vi "SimpleOscilloscopeMain.vi"() -> ()   [LabVIEW 2020]
uses:
  Oscilloscope.lvclass
  Oscilloscope.lvclass/Oscilloscope.ctl
panel:
  out "Waveform Graph":waveform(dbl)[](graph)
  out "error out":errorcluster
  in  "Stop Button":bool
  in  "error in (no error)":errorcluster
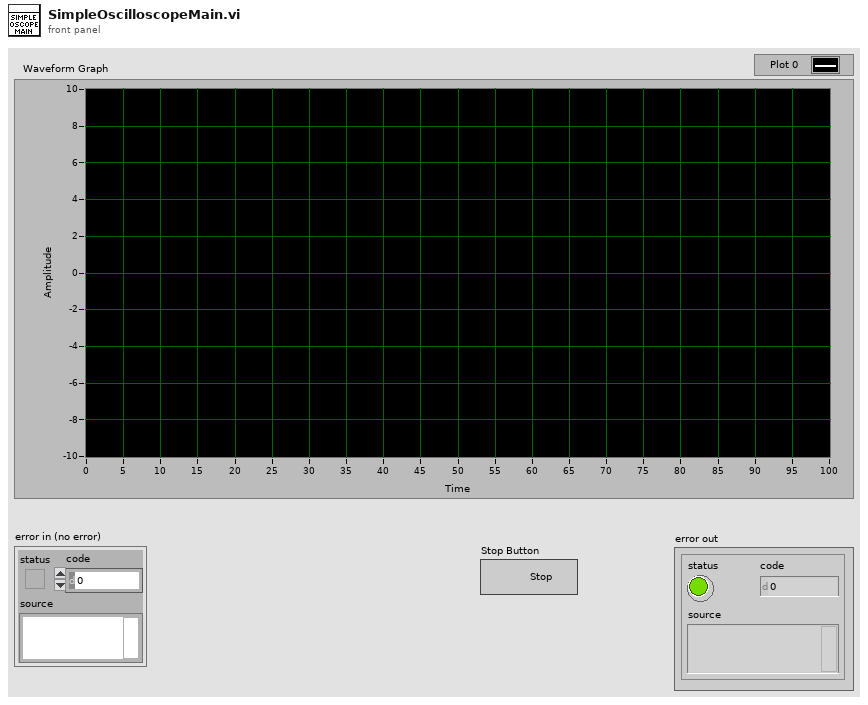
[diagram p1: front panel]
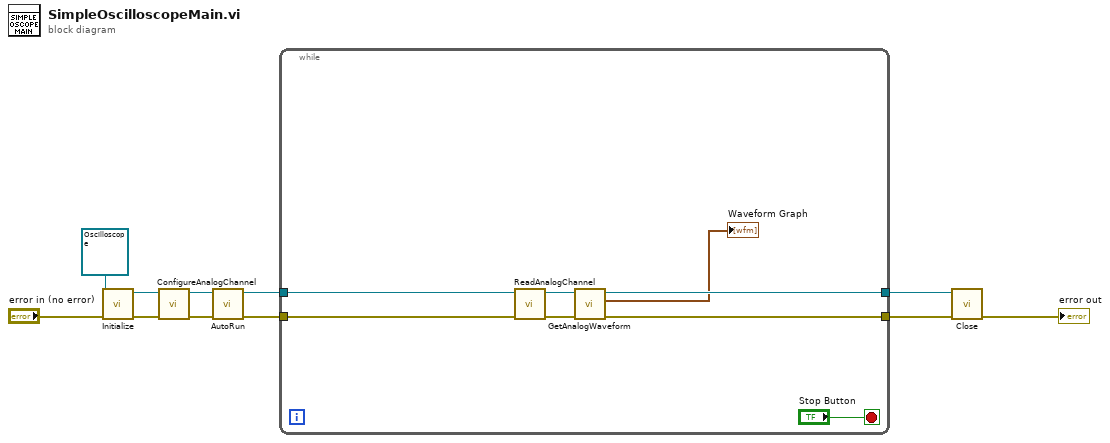
[diagram p0: block diagram]
diagram:
  n1 = call-dynamic "Initialize.vi"("error in (no error)"="error in (no error)", "Oscilloscope in"=refnum<class "Oscilloscope.lvclass"> refnum) -> ("error out"=w9:errorcluster, "Oscilloscope out"=w7:refnum<class "Oscilloscope.lvclass">)  [unwired: 8 in]
  n2 = call "ConfigureAnalogChannel.vi"("error in (no error)"=w9, "Oscilloscope in"=w7) -> ("error out"=w8:errorcluster, "Oscilloscope out"=w6:refnum<class "Oscilloscope.lvclass">)  [unwired: 8 in]
  n3 = call "AutoRun.vi"("error in (no error)"=w8, "Oscilloscope in"=w6) -> ("error out"=w5:errorcluster, "Oscilloscope out"=w4:refnum<class "Oscilloscope.lvclass">)  [unwired: 8 in]
  n4 = while {
    tunnel: w5 -> [w19]
    tunnel: w4 -> [w18]
    tunnel: [w15] -> w3
    tunnel: [w13] -> w2
    stop <- "Stop Button" stop-if-true
    n5 = call "ReadAnalogChannel.vi"("error in (no error)"=w19, "Oscilloscope in"=w18) -> ("error out"=w17:errorcluster, "Oscilloscope out"=w16:refnum<class "Oscilloscope.lvclass">)  [unwired: 8 in]
    n6 = call "GetAnalogWaveform.vi"("error in (no error)"=w17, "Oscilloscope in"=w16) -> ("error out"=w15:errorcluster, "AnalogWaveform"=→"Waveform Graph":waveform(dbl)[], "Oscilloscope out"=w13:refnum<class "Oscilloscope.lvclass">)  [unwired: 7 in]
  }
  n7 = call-dynamic "Close.vi"("error in (no error)"=w3, "Oscilloscope in"=w2) -> ("error out"=→"error out":errorcluster)  [unwired: 8 in, 1 out]
